vi "WindowBuild.vi"(7 "Init":bool, 8 "error in (no error)":errorcluster, 11 "Fitter in":refnum<class "FitterBase.lvclass">) -> (0 "error out":errorcluster, 2 "Timeout":bool, 3 "Fitter out":refnum<class "FitterBase.lvclass">)   [LabVIEW 2018, in "AnalysisPlugins.lvlib" / "FitterBase.lvclass"]
uses:
  FitterBaseClass/FitterBase.lvclass
  X:/Projects/PMUCal/Modules/Analysis/AnalysisPlugins/AnalysisPluginBaseClass/AnalysisPluginsBase.lvclass
  Typedefs/SampleDataInput.ctl
  FitterBaseClass/Typedefs/clAnalysisConfig.ctl
  AnalysisPluginsBase.lvclass/AnalysisPluginsBase.ctl
  FitterBaseClass/Typedefs/Wvfrm_ref.ctl
  Accessors/Read SensorQue.vi
  Accessors/Read Duration.vi
  Accessors/Read Window.vi
  Accessors/Read AnalysisConfig.vi
  Accessors/Read AnalysisTime.vi
  Accessors/Read SampleDataQueName.vi
  Accessors/Write Window.vi
  <vilib>/Utility/error.llb/Error Cluster From Error Code.vi
  <vilib>/ErrorRing/Error Ring.xnode
  AnalysisPluginsBase.lvclass
panel:
  out "T0":timestamp format="%^<%.3X\n%x>T"
  out "Continue":bool
  out "Valid":bool
  out "SensorTime":timestamp format="%^<%.3X\n%x>T"
  out "WindowTime":timestamp format="%^<%.3X\n%x>T"
  out "SampleTime":timestamp format="%^<%.3X\n%x>T"
  out "SampleData":dbl[][](graph)
  out "Window":dbl[][](graph)
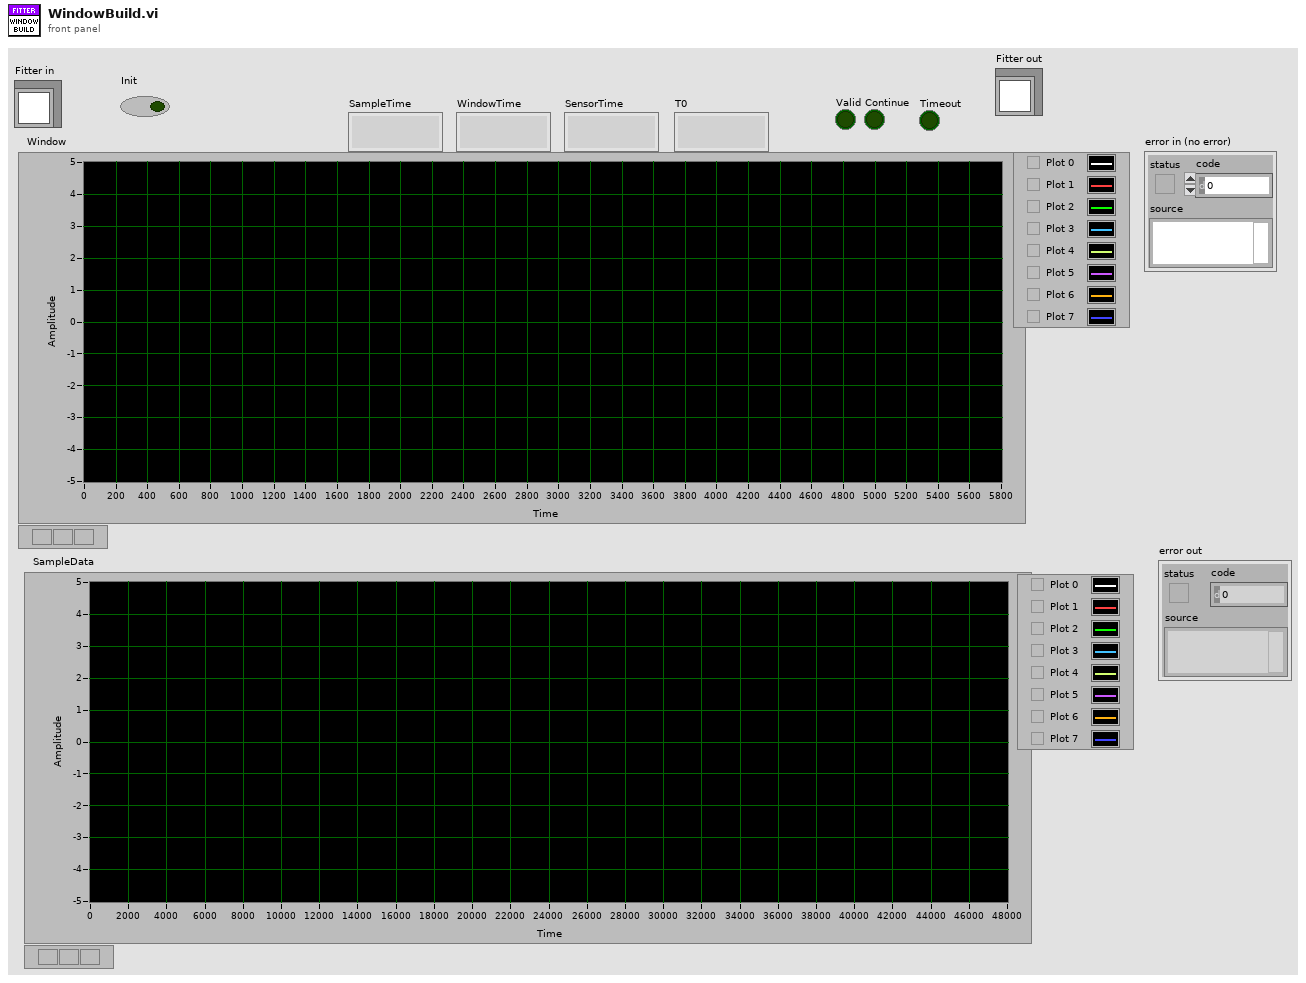
[diagram p1: front panel]
types:
  T1 = typedef "AnalysisPlugins.lvlib/FitterBase.lvclass/clAnalysisConfig.ctl" = cluster{"F0":u32, "SettlingTime":dbl, "AnalysisCycles":dbl, "SampleRate":dbl, "NumChannels":u32, "TsOffset":enum16{"start", "middle", "end"}}
  T2 = typedef "AnalysisPlugins.lvlib/AnalysisPluginsBase.lvclass/SampleDataInput.ctl" = waveform(dbl)[]
  T3 = typedef "AnalysisPlugins.lvlib/FitterBase.lvclass/Wvfrm_ref.ctl" = cluster{"t0":timestamp, "dt":dbl, "attributes":variant, "Y_ref":refnum<data-value>}
  T4 = typedef "AnalysisPlugins.lvlib/AnalysisPluginsBase.lvclass/clWindowData.ctl" = cluster{"Timestamp":ext, "Samples":dbl[][], "Window Valid":bool, "T0":ext}
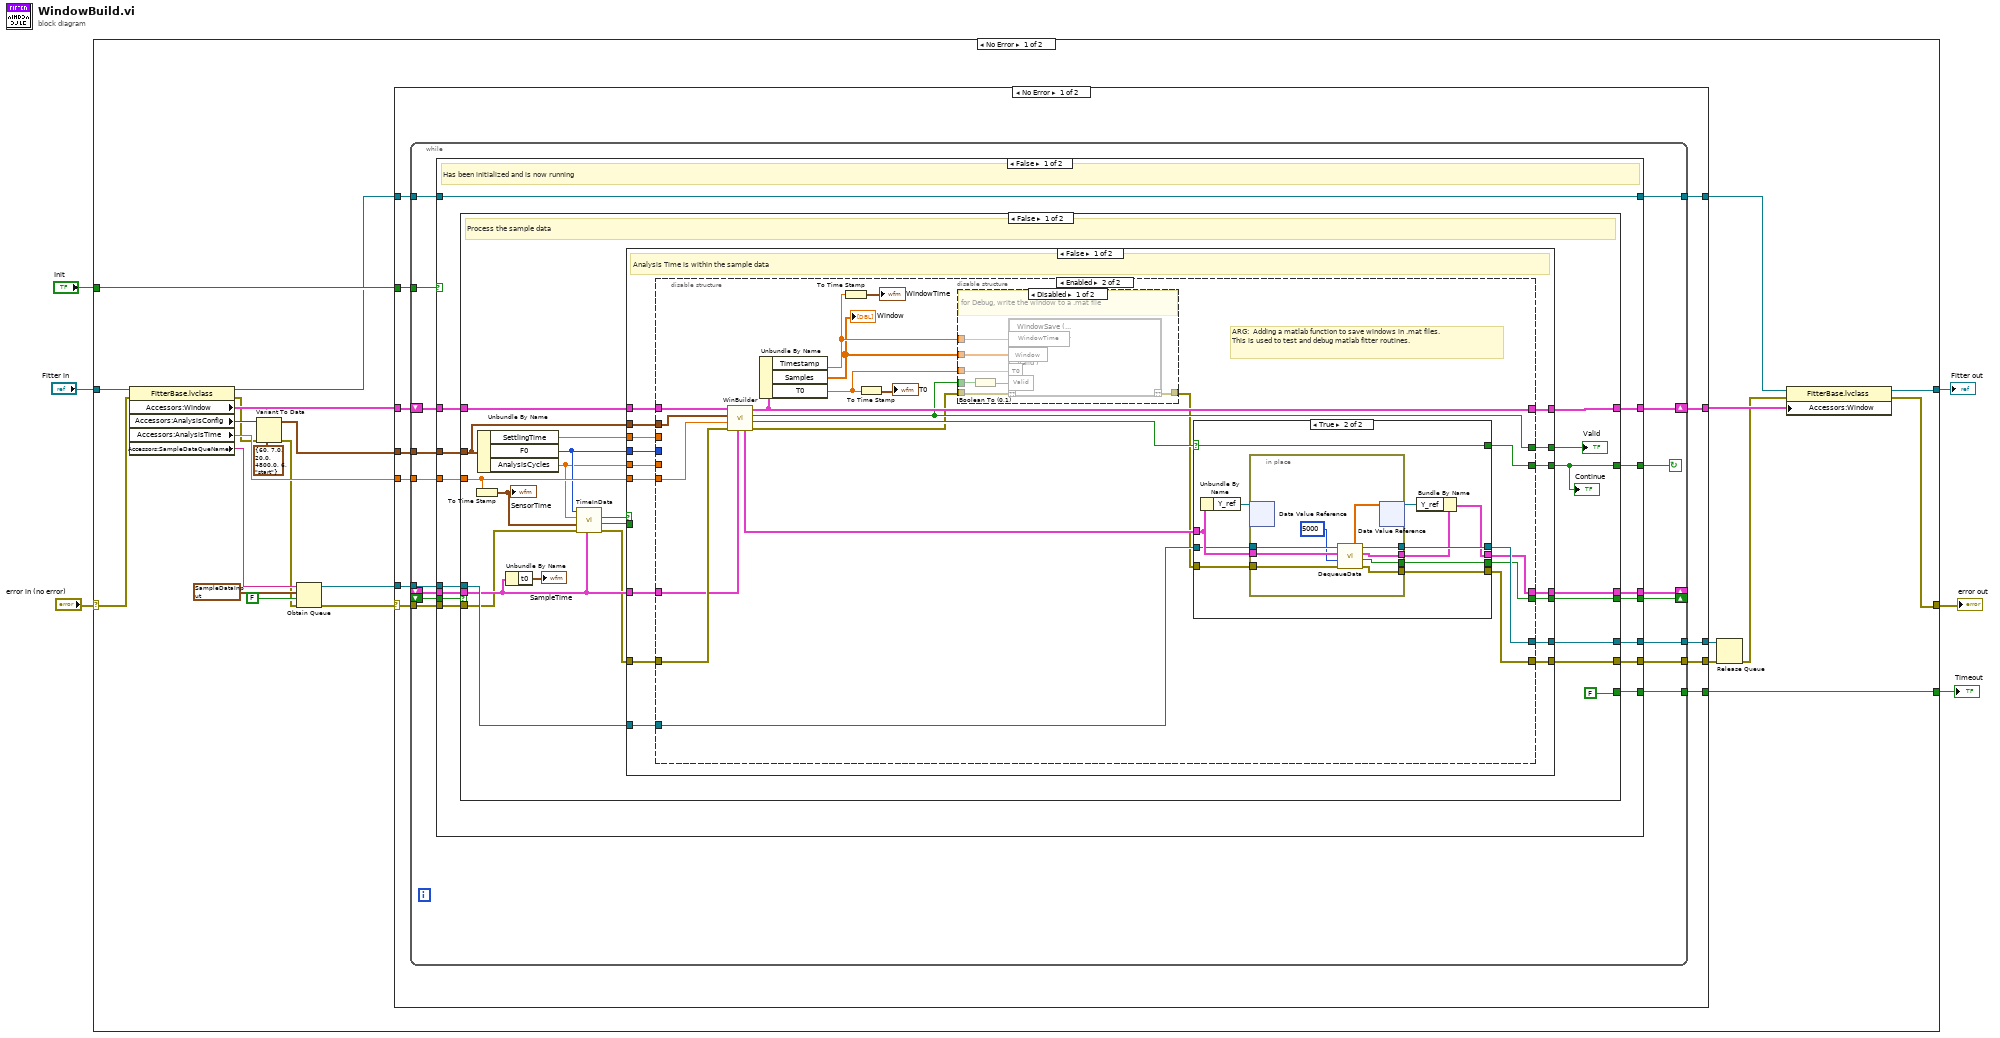
[diagram p0: block diagram]
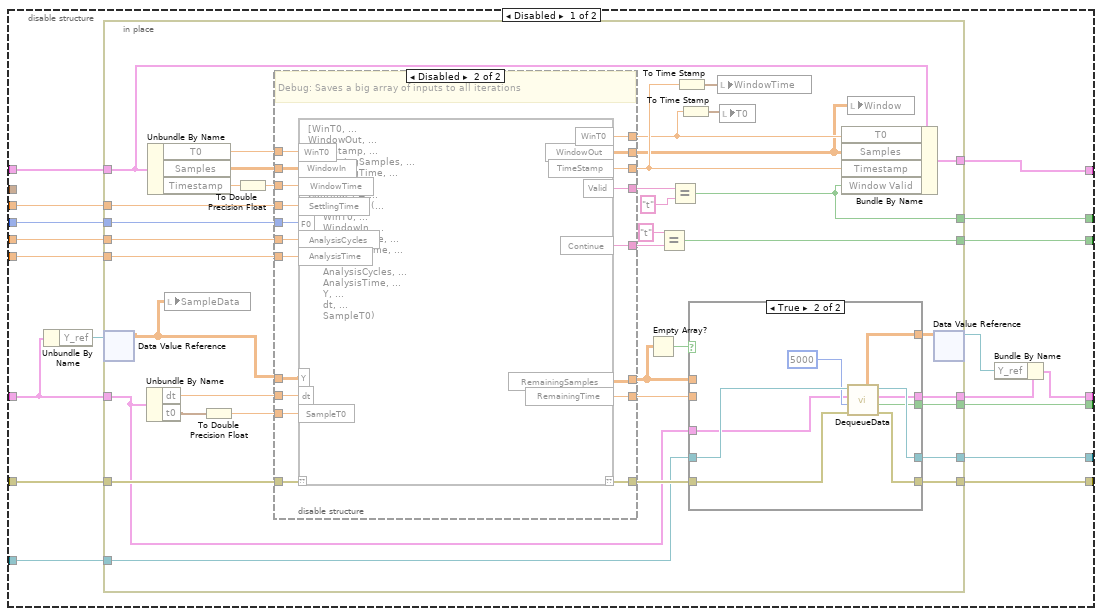
[diagram p2: hidden frame]
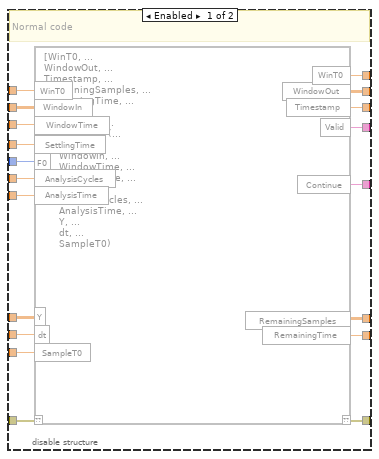
[diagram p3: hidden frame]
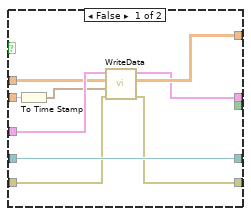
[diagram p4: hidden frame]
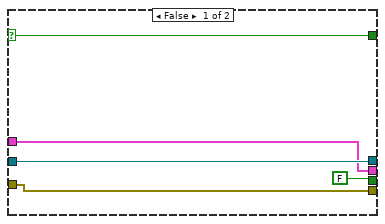
[diagram p6: hidden frame]
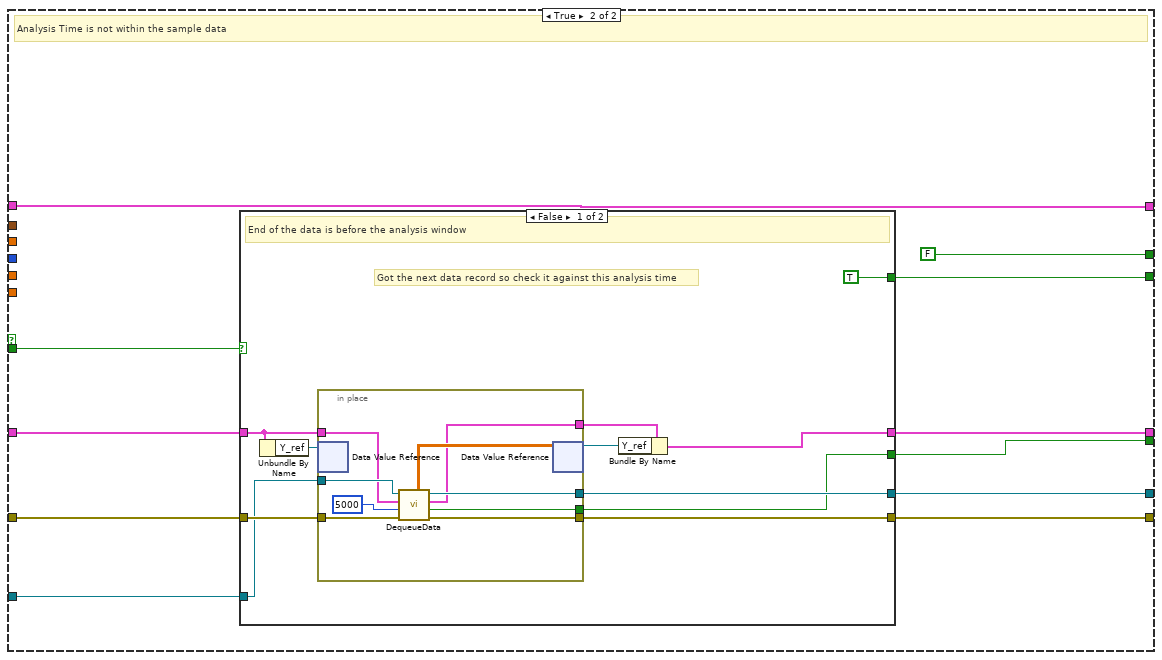
[diagram p7: hidden frame]
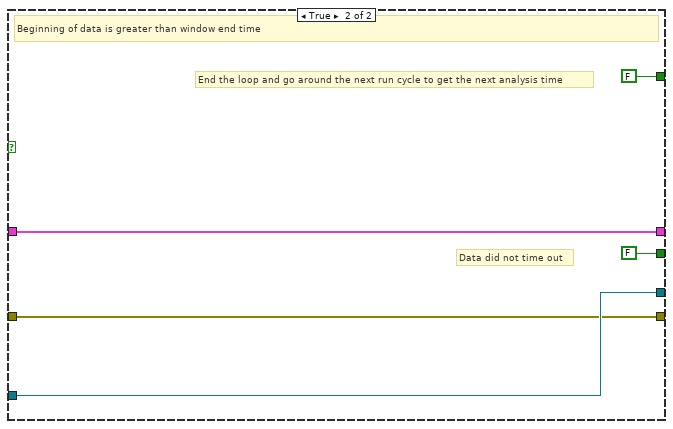
[diagram p8: hidden frame]
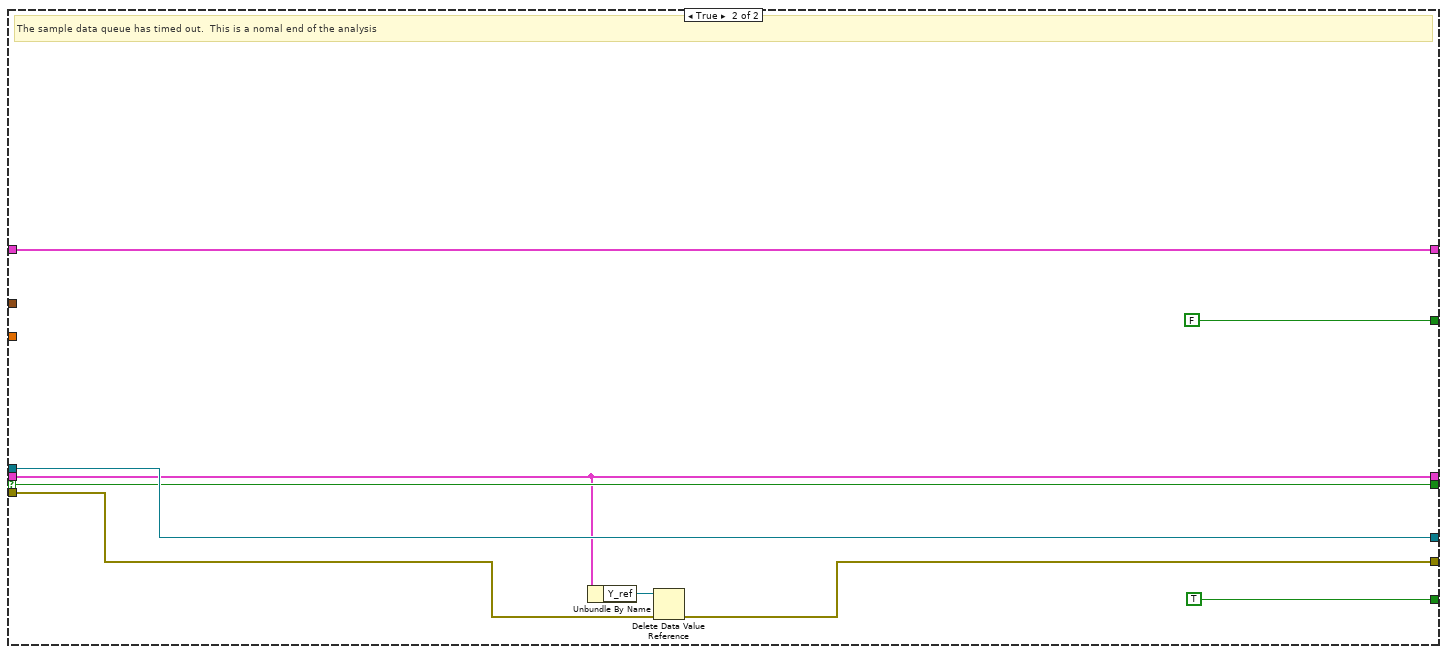
[diagram p9: hidden frame]
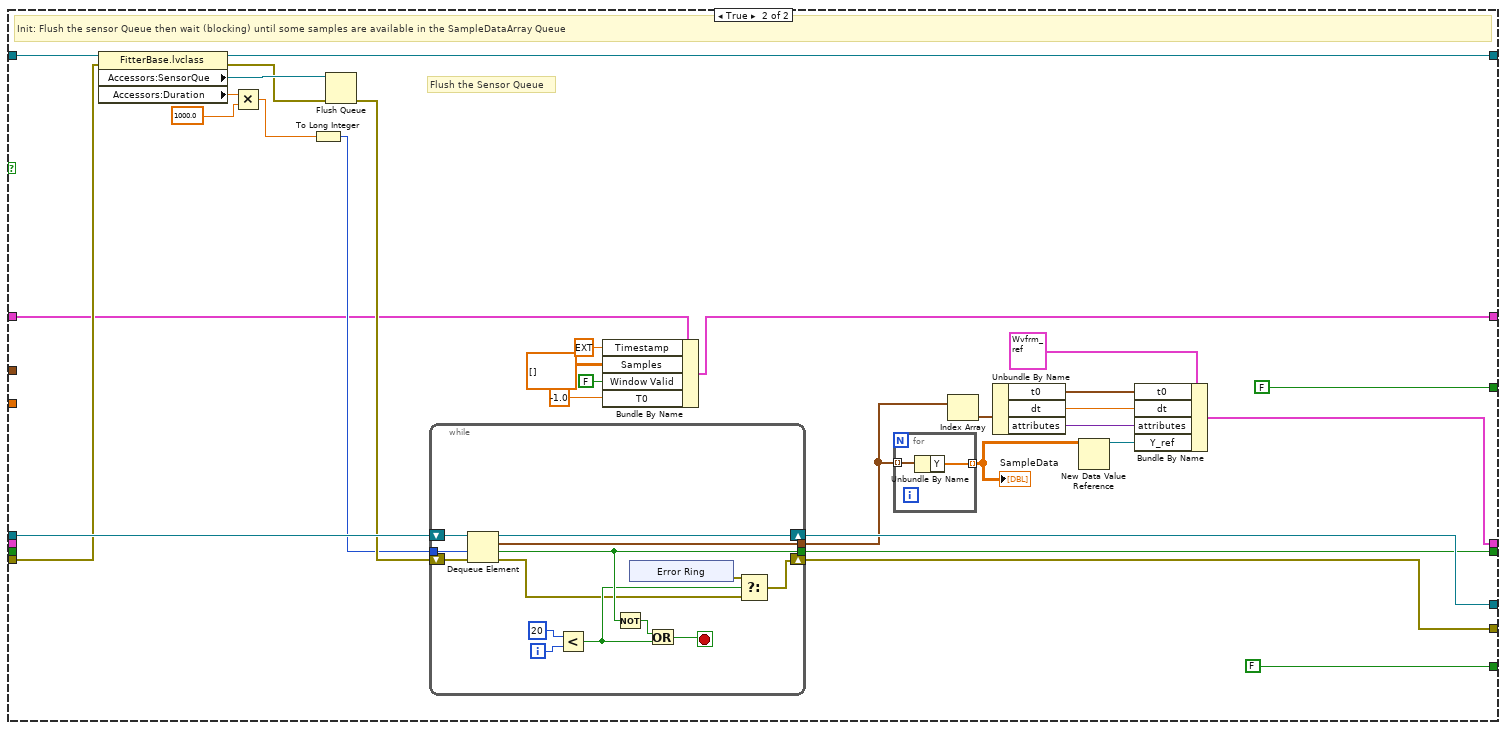
[diagram p10: hidden frame]
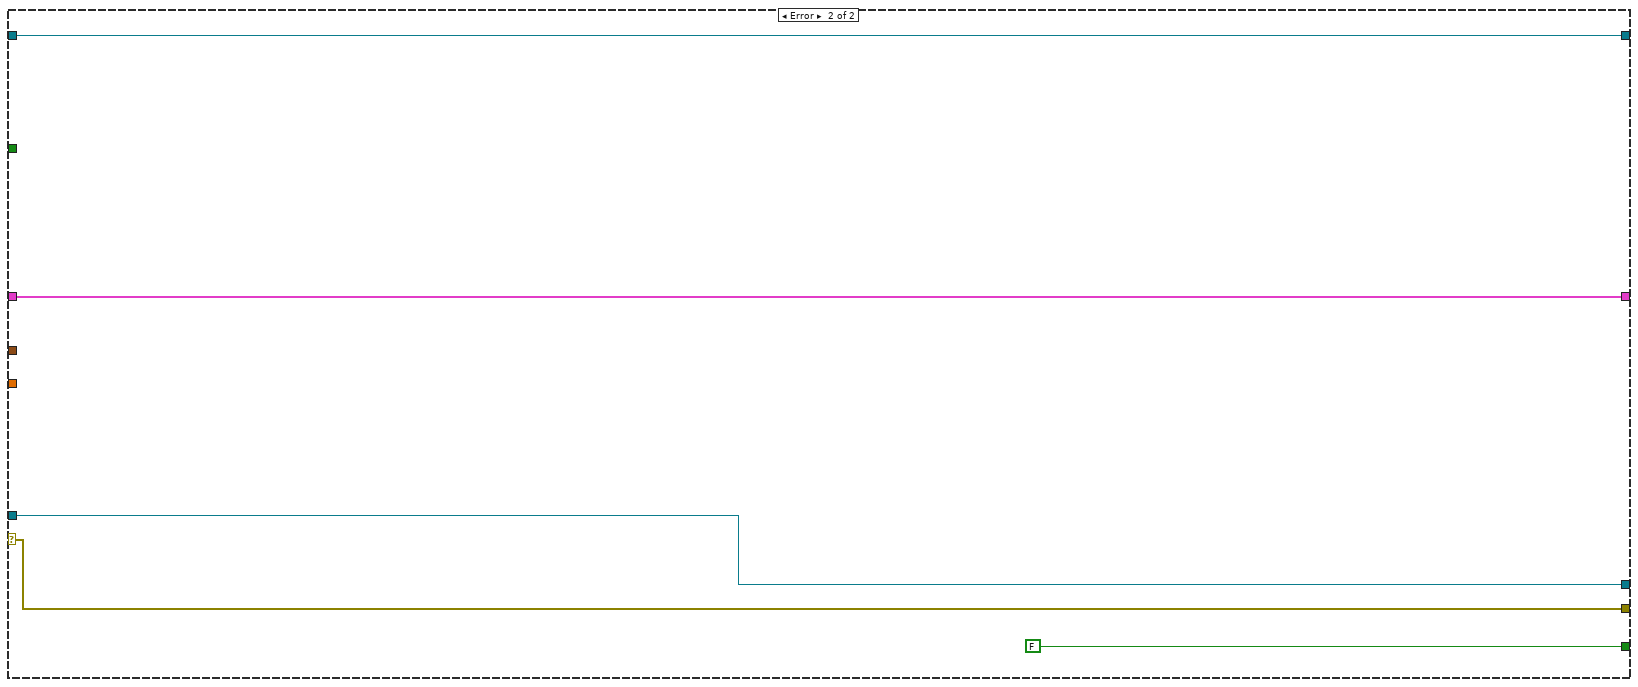
[diagram p11: hidden frame]
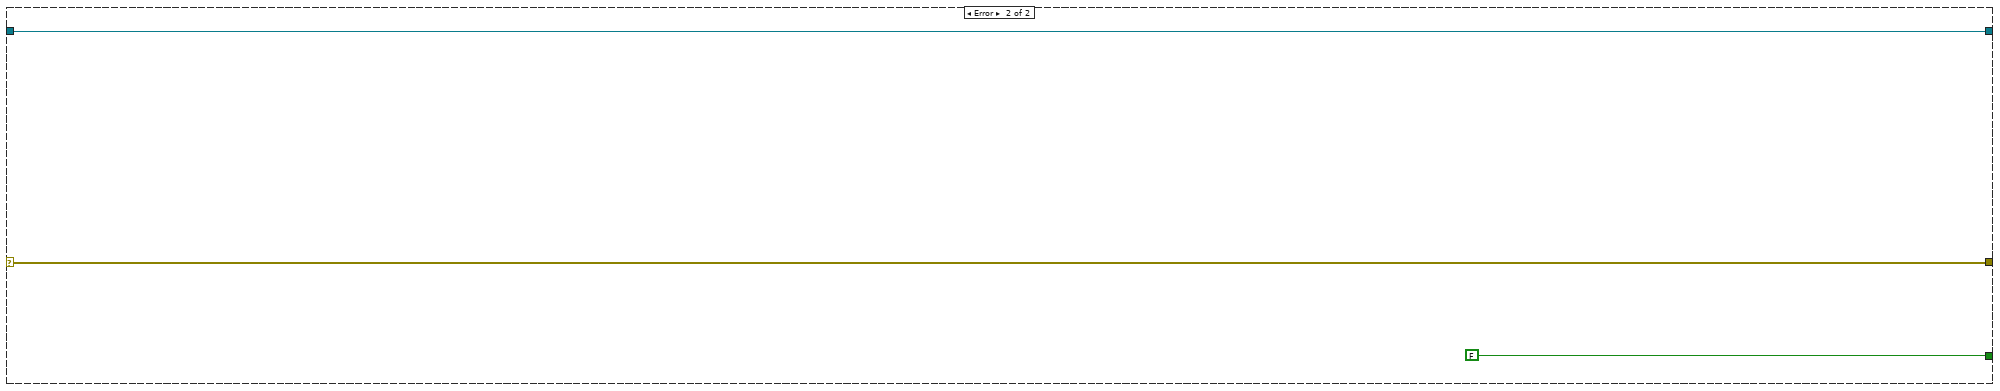
[diagram p12: hidden frame]
diagram:
  n1 = case shown="No Error" "error in (no error)" {
    selector: "error in (no error)" -> [w15 w382]
    tunnel: [w28 w382] -> w5
    tunnel: [w29 w381] -> w3
    tunnel: "Fitter in" -> [w30 w381]
    tunnel: [w18 FALSE] -> w2
    tunnel: "Init" -> [w10 _]
    frame No Error {
      n2 = property class="FitterBase.lvclass"(reference=w30, error in=w15) -> (reference out=w9:refnum<class "FitterBase.lvclass">, error out=w14:errorcluster, "Accessors:Window"=w24:T4, "Accessors:AnalysisConfig"=w17:variant, "Accessors:AnalysisTime"=w25:dbl, "Accessors:SampleDataQueName"=w26:string)
      n3 = Variant To Data(error in=w14, type=T1 {"F0"=60, "SettlingTime"=7.0, "AnalysisCycles"=20.0, "SampleRate"=4800.0, "NumChannels"=6, "TsOffset"=enum."start"} ("clAnalysisConfig"), Variant=w17) -> (data=w7:T1, error out=w13:errorcluster)
      n4 = Obtain Queue(name (unnamed)=w26, element data type=T2 [{"t0"=timestamp(0 s since 1904-01-01), "dt"=1.0, "Y"=[]}] ("clSampleDataArray"), create if not found? (T)=FALSE, error in (no error)=w13) -> (queue out=w12:refnum<queue>, error out=w11:errorcluster)  [unwired: 1 in, 1 out]
      n5 = case shown="No Error" w11 {
        selector: w11 -> [w41 w379]
        tunnel: w25 -> [w42 _]
        tunnel: w12 -> [w40 w378]
        tunnel: w24 -> [w39 w377]
        tunnel: [w38 w377] -> w23
        tunnel: [w37 w379] -> w22
        tunnel: [w36 w378] -> w20
        tunnel: [w35 FALSE] -> w18
        tunnel: w10 -> [w34 _]
        tunnel: w9 -> [w33 w375]
        tunnel: [w32 w375] -> w8
        tunnel: w7 -> [w31 _]
        frame No Error {
          n6 = while {
            tunnel: w42 -> [w59]
            tunnel: w41 -> [w55]
            tunnel: w40 -> [w53]
            shift-right: [w56] -> w38
            shift-left: w39 -> [w57]
            tunnel: [w54] -> w37
            tunnel: [w52] -> w36
            tunnel: [w51] -> w35
            shift-right: [w44] -> _
            shift-left: _ -> [w50]
            shift-right: [w48] -> _
            shift-left: _ -> [w49]
            tunnel: w34 -> [w47]
            tunnel: w33 -> [w46]
            tunnel: [w45] -> w32
            tunnel: w31 -> [w43]
            stop <- w58 continue-if-true
            n7 = case shown="False" w47 {
              tunnel: w50 -> [w61 _]
              tunnel: w59 -> [w74 _]
              tunnel: [w73 FALSE] -> w58
              tunnel: w57 -> [w72 w329]
              tunnel: [w71 w324] -> w56
              tunnel: w49 -> [w70 _]
              tunnel: w55 -> [w69 w345]
              tunnel: [w68 w341] -> w54
              tunnel: w53 -> [w67 w354]
              tunnel: [w66 w353] -> w52
              tunnel: [w65 FALSE] -> w51
              tunnel: [w64 w335] -> w44
              tunnel: [w63 w352] -> w48
              tunnel: w46 -> [w62 w349]
              tunnel: [w62 w346] -> w45
              tunnel: w43 -> [w60 _]
              frame False {
                # "Has been initialized and is now running"
                n8 = case shown="False" w70 {
                  selector: w70 -> [_ w319]
                  tunnel: w74 -> [w89 _]
                  tunnel: [w96 FALSE] -> w73
                  tunnel: w72 -> [w95 w322]
                  tunnel: [w94 w322] -> w71
                  tunnel: w69 -> [w76 w318]
                  tunnel: [w91 w317] -> w68
                  tunnel: w67 -> [w92 w321]
                  tunnel: [w90 w321] -> w66
                  tunnel: [FALSE TRUE] -> w65
                  tunnel: [w81 w316] -> w64
                  tunnel: [w87 w319] -> w63
                  tunnel: w61 -> [w82 w316]
                  tunnel: w60 -> [w77 _]
                  frame False {
                    # "Process the sample data"
                    n9 = To Time Stamp(1:w89) -> (0:w86:timestamp)
                    "SensorTime" <- w86
                    n10 = Unbundle By Name(w77) -> ("SettlingTime"=w80:dbl, "F0"=w79:u32, "AnalysisCycles"=w78:dbl)
                    n11 = Unbundle By Name(w82) -> ("t0"=→"SampleTime":timestamp)
                    n12 = call "TimeInData.vi"("Wvfrm_ref"=w82, "error in (no error)"=w76, "SensorTime"=w86, "AnalysisCycles"=w78, "F0"=w79) -> ("error out"=w75:errorcluster, "AnalysisFirst"=w84:bool, "NoDataInWindow"=w85:bool)  [unwired: 4 in]
                    n13 = case shown="False" w85 {
                      tunnel: w79 -> [w112 _]
                      tunnel: w78 -> [w111 _]
                      tunnel: [w110 w280] -> w96
                      tunnel: w95 -> [w109 w289]
                      tunnel: [w108 w289] -> w94
                      tunnel: [w107 FALSE] -> w93
                      tunnel: w92 -> [w106 w284]
                      tunnel: [w105 w281] -> w91
                      tunnel: [w104 w283] -> w90
                      tunnel: w75 -> [w103 w282]
                      tunnel: w89 -> [w102 _]
                      tunnel: w80 -> [w101 _]
                      tunnel: [w98 w279] -> w81
                      tunnel: [w100 w285] -> w87
                      tunnel: w82 -> [w99 w286]
                      tunnel: w84 -> [_ w287]
                      tunnel: w77 -> [w97 _]
                      frame False {
                        # "Analysis Time is within the sample data"
                        n14 = disable-structure shown="Enabled" {
                          disable-tunnel: w112 -> [w130 _]
                          disable-tunnel: w111 -> [w129 _]
                          disable-tunnel: [w128 w231] -> w110
                          disable-tunnel: w109 -> [w127 w245]
                          disable-tunnel: [w126 w240] -> w108
                          disable-tunnel: [w125 w227] -> w107
                          disable-tunnel: w106 -> [w124 w234]
                          disable-tunnel: [w123 w232] -> w105
                          disable-tunnel: [w122 w235] -> w104
                          disable-tunnel: w103 -> [w121 w243]
                          disable-tunnel: w102 -> [w120 w242]
                          disable-tunnel: w101 -> [w119 _]
                          disable-tunnel: [w118 w230] -> w100
                          disable-tunnel: w99 -> [w117 w241]
                          disable-tunnel: [w113 w233] -> w98
                          disable-tunnel: w97 -> [_ w244]
                          frame Disabled {
                            n15 = Unbundle By Name(w117) -> ("Y_ref"=w116:refnum<data-value>)
                            n16 = in-place {
                              in-place-border: w130 -> [w167]
                              in-place-border: w129 -> [w166]
                              in-place-border: [w165] -> w128
                              in-place-border: w127 -> [w164]
                              in-place-border: [w163] -> w126
                              in-place-border: [w157] -> w125
                              in-place-border: w124 -> [w154]
                              in-place-border: [w153] -> w123
                              in-place-border: [w151] -> w122
                              in-place-border: w121 -> [w150]
                              in-place-border: w120 -> [w148]
                              in-place-border: w119 -> [w146]
                              in-place-border: [w144] -> w118
                              in-place-border: w117 -> [w142]
                              in-place-border: [w143] -> w115
                              n17 = in-place-dvr #1(w116) -> (w136:dbl[][])  [unwired: 1 out]
                              n18 = Unbundle By Name(w142) -> ("dt"=w139:dbl, "t0"=w138:timestamp)
                              n19 = Unbundle By Name(w164) -> ("T0"=w145:ext, "Samples"=w162:dbl[][], "Timestamp"=w149:ext)
                              n20 = local write "SampleData"(w136) -> ()
                              n21 = To Double Precision Float(number=w138) -> (double precision float=w137:dbl)
                              n22 = To Double Precision Float(number=w149) -> (double precision float=w156:dbl)
                              n23 = disable-structure shown="Disabled" {
                                disable-tunnel: w167 -> [w186 w203]
                                disable-tunnel: w166 -> [w185 w202]
                                disable-tunnel: w148 -> [w184 w201]
                                disable-tunnel: w162 -> [w183 w205]
                                disable-tunnel: [w182 w196] -> w161
                                disable-tunnel: [w181 w199] -> w131
                                disable-tunnel: [w180 w198] -> w134
                                disable-tunnel: [w179 w197] -> w159
                                disable-tunnel: w150 -> [w178 w193]
                                disable-tunnel: w136 -> [w177 w200]
                                disable-tunnel: w156 -> [w176 w204]
                                disable-tunnel: [w175 w194] -> w155
                                disable-tunnel: [w174 w195] -> w147
                                disable-tunnel: w146 -> [w172 w192]
                                disable-tunnel: w145 -> [w173 w191]
                                disable-tunnel: [w171 w190] -> w132
                                disable-tunnel: [w170 w189] -> w140
                                disable-tunnel: w139 -> [w169 w187]
                                disable-tunnel: w137 -> [w168 w188]
                                frame Enabled {
                                # "Normal code"
                                n24 = script code="[WinT0, ...\nWindowOut, ...\nTimestamp, ...\nRemainingSamples, ...\nRemainingTime, ...\nValid, ...\nContinue] = ...\nWindowBuild (...\n     WinT0, ...\n     WindowIn, ...\n     WindowTime, ...\n     SettlingTime, ...\n      F0, ...\n     AnalysisCycles, ...\n     AnalysisTime, ...\n     Y, ...\n     dt, ...\n     SampleT0)"("??"=w178, "F0"=w186, "AnalysisCycles"=w185, "AnalysisTime"=w184, "WindowTime"=w176, "Y"=w177, "dt"=w169, "SampleT0"=w168, "WindowIn"=w183, "WinT0"=w173, "SettlingTime"=w172) -> ("??"=w175:errorcluster, "Continue"=w182:string, "WindowOut"=w181:dbl[][], "Timestamp"=w180:dbl, "Valid"=w179:string, "RemainingSamples"=w174:dbl[][], "RemainingTime"=w170:dbl, "WinT0"=w171:dbl)
                                }
                                frame Disabled {
                                # "Debug: Saves a big array of inputs to all iterations"
                                n25 = script code="[WinT0, ...\nWindowOut, ...\nTimeStamp, ...\nRemainingSamples, ...\nRemainingTime, ...\nValid, ...\nContinue] = ...\nWindowSave (...\n     WinT0, ...\n     WindowIn, ...\n     WindowTime, ...\n      SettlingTime, ...\n      F0, ...\n     AnalysisCycles, ...\n     AnalysisTime, ...\n     Y, ...\n     dt, ...\n     SampleT0)"("??"=w193, "F0"=w203, "AnalysisCycles"=w202, "AnalysisTime"=w201, "WindowTime"=w204, "Y"=w200, "dt"=w187, "SampleT0"=w188, "WindowIn"=w205, "SettlingTime"=w192, "WinT0"=w191) -> ("??"=w194:errorcluster, "Continue"=w196:string, "WindowOut"=w199:dbl[][], "TimeStamp"=w198:dbl, "Valid"=w197:string, "RemainingSamples"=w195:dbl[][], "RemainingTime"=w189:dbl, "WinT0"=w190:dbl)
                                }
                              }
                              n26 = Empty Array?(array=w147) -> (empty?=w152:bool)
                              n27 = Equal?(x="t", y=w161) -> (x = y?=w165:bool)
                              n28 = Equal?(x=w159, y="t") -> (x = y?=w157:bool)
                              n29 = To Time Stamp(1:w134) -> (0:w135:timestamp)
                              n30 = To Time Stamp(1:w132) -> (0:w133:timestamp)
                              n31 = case shown="True" w152 {
                                tunnel: w155 -> [w208 w220]
                                tunnel: w154 -> [w214 w223]
                                tunnel: [w207 w218] -> w153
                                tunnel: [w214 w222] -> w151
                                tunnel: w147 -> [w211 _]
                                tunnel: [w209 w221] -> w143
                                tunnel: [_ w219] -> w144
                                tunnel: w142 -> [w212 w216]
                                tunnel: [w210 w215] -> w141
                                tunnel: w140 -> [w213 _]
                                frame False {
                                n32 = To Time Stamp(1:w213) -> (0:w206:timestamp)
                                n33 = call "WriteData.vi"("error in (no error)"=w208, "t0"=w206, "data value"=w211, "Wvfrm_ref"=w212) -> ("error out"=w207:errorcluster, "data value"=w210:dbl[][], "Wvfrm_ref"=w209:T3)  [unwired: 5 in]
                                }
                                frame True {
                                n34 = call "DequeueData.vi"("error in (no error)"=w220, "timeout in ms (-1)"=5000, "DataIn"=w216, "queue in"=w223) -> ("error out"=w218:errorcluster, "timed out?"=w219:bool, "Data Out"=w221:T3, "queue out"=w222:refnum<queue>, "Y"=w215:dbl[][])  [unwired: 3 in]
                                }
                              }
                              n35 = local write "WindowTime"(w135) -> ()
                              n36 = local write "T0"(w133) -> ()
                              n37 = Bundle By Name(cluster=w164, "T0"=w132, "Samples"=w131, "Timestamp"=w134, "Window Valid"=w157) -> (w163:T4)
                              n38 = local write "Window"(w131) -> ()
                              n39 = in-place-dvr #1(w141) -> (w114:refnum<data-value>)  [unwired: 1 out]
                            }
                            n40 = Bundle By Name(cluster=w115, "Y_ref"=w114) -> (w113:T3)
                          }
                          frame Enabled {
                            # "ARG:  Adding a matlab function to save windows in .mat files.\nThis is used to test and debug matlab fitter routines."
                            n41 = call "WinBuilder.vi"("Wvfrm_ref"=w241, "error in (no error)"=w243, "AnalysisTime"=w242, "clAnalysisConfig"=w244, "Window"=w245) -> ("error out"=w225:errorcluster, "Continue"=w237:bool, "Valid"=w227:bool, "Window"=w240:T4, "Wvfrm_ref"=w236:T3)  [unwired: 2 in]
                            n42 = Unbundle By Name(w240) -> ("Timestamp"=w229:ext, "Samples"=w228:dbl[][], "T0"=w226:ext)
                            "Window" <- w228
                            n43 = To Time Stamp(1:w229) -> (0:→"WindowTime":timestamp)
                            n44 = To Time Stamp(1:w226) -> (0:→"T0":timestamp)
                            n45 = disable-structure shown="Disabled" {
                              disable-tunnel: w225 -> [w252 w253]
                              disable-tunnel: w229 -> [w251 _]
                              disable-tunnel: w228 -> [w250 _]
                              disable-tunnel: w227 -> [w249 _]
                              disable-tunnel: w226 -> [w247 _]
                              disable-tunnel: [w246 w253] -> w224
                              frame Disabled {
                                # "for Debug, write the window to a .mat file"
                                n46 = Boolean To (0,1)(Boolean=w249) -> (0, 1=w248:i16)
                                n47 = script code="WindowSave (...\nWindowTime, ...\nWindow, ...\nT0, ...\nValid )"("??"=w252, "WindowTime"=w251, "Window"=w250, "T0"=w247, "Valid"=w248) -> ("??"=w246:errorcluster)
                              }
                              frame Enabled {
                              }
                            }
                            n48 = case shown="True" w237 {
                              selector: w237 -> [w255 w263]
                              tunnel: w234 -> [w258 w267]
                              tunnel: w236 -> [w257 w269]
                              tunnel: w224 -> [w256 w266]
                              tunnel: [w258 w265] -> w235
                              tunnel: [w257 w260] -> w233
                              tunnel: [w256 w264] -> w232
                              tunnel: [w255 w263] -> w231
                              tunnel: [FALSE w262] -> w230
                              frame False {
                              }
                              frame True {
                                n49 = Unbundle By Name(w269) -> ("Y_ref"=w268:refnum<data-value>)
                                n50 = in-place {
                                in-place-border: w269 -> [w277]
                                in-place-border: w267 -> [w278]
                                in-place-border: w266 -> [w275]
                                in-place-border: [w273] -> w265
                                in-place-border: [w272] -> w261
                                in-place-border: [w271] -> w262
                                in-place-border: [w270] -> w264
                                n51 = in-place-dvr #2(w268) -> ()  [unwired: 2 out]
                                n52 = call "DequeueData.vi"("error in (no error)"=w275, "timeout in ms (-1)"=5000, "DataIn"=w277, "queue in"=w278) -> ("error out"=w270:errorcluster, "timed out?"=w271:bool, "Data Out"=w272:T3, "queue out"=w273:refnum<queue>, "Y"=w274:dbl[][])  [unwired: 3 in]
                                n53 = in-place-dvr #2(w274) -> (w259:refnum<data-value>)  [unwired: 1 out]
                                }
                                n54 = Bundle By Name(cluster=w261, "Y_ref"=w259) -> (w260:T3)
                              }
                            }
                          }
                        }
                      }
                      frame True {
                        # "Analysis Time is not within the sample data"
                        n55 = case shown="False" w287 {
                          tunnel: w286 -> [w294 w314]
                          tunnel: [w290 w314] -> w279
                          tunnel: [w295 FALSE] -> w285
                          tunnel: w284 -> [w298 w312]
                          tunnel: [w297 w312] -> w283
                          tunnel: w282 -> [w299 w311]
                          tunnel: [w296 w311] -> w281
                          tunnel: [TRUE FALSE] -> w280
                          frame False {
                            # "Got the next data record so check it against this analysis time"
                            # "End of the data is before the analysis window"
                            n56 = Unbundle By Name(w294) -> ("Y_ref"=w293:refnum<data-value>)
                            n57 = in-place {
                              in-place-border: w299 -> [w309]
                              in-place-border: w298 -> [w307]
                              in-place-border: w294 -> [w306]
                              in-place-border: [w305] -> w297
                              in-place-border: [w304] -> w296
                              in-place-border: [w303] -> w295
                              in-place-border: [w301] -> w292
                              n58 = in-place-dvr #3(w293) -> ()  [unwired: 2 out]
                              n59 = call "DequeueData.vi"("error in (no error)"=w309, "timeout in ms (-1)"=5000, "DataIn"=w306, "queue in"=w307) -> ("error out"=w304:errorcluster, "timed out?"=w303:bool, "Data Out"=w301:T3, "queue out"=w305:refnum<queue>, "Y"=w302:dbl[][])  [unwired: 3 in]
                              n60 = in-place-dvr #3(w302) -> (w291:refnum<data-value>)  [unwired: 1 out]
                            }
                            n61 = Bundle By Name(cluster=w292, "Y_ref"=w291) -> (w290:T3)
                          }
                          frame True {
                            # "End the loop and go around the next run cycle to get the next analysis time"
                            # "Data did not time out"
                            # "Beginning of data is greater than window end time"
                          }
                        }
                      }
                    }
                    "Valid" <- w93
                    "Continue" <- w96
                  }
                  frame True {
                    # "The sample data queue has timed out.  This is a nomal end of the analysis"
                    n62 = Unbundle By Name(w316) -> ("Y_ref"=w315:refnum<data-value>)
                    n63 = Delete Data Value Reference(data value reference=w315, error in=w318) -> (error out=w317:errorcluster)  [unwired: 1 out]
                  }
                }
              }
              frame True {
                # "Flush the Sensor Queue"
                # "Init: Flush the sensor Queue then wait (blocking) until some samples are available in the SampleDataArray Queue"
                n64 = property class="FitterBase.lvclass"(reference=w349, error in=w345) -> (reference out=w346:refnum<class "FitterBase.lvclass">, error out=w347:errorcluster, "Accessors:SensorQue"=w348:refnum<queue>, "Accessors:Duration"=w344:dbl)
                n65 = Multiply(x=w344, y=1000.0) -> (x*y=w330:dbl)
                n66 = To Long Integer(number=w330) -> (32bit integer=w331:i32)
                n67 = Flush Queue(queue=w348, error in (no error)=w347) -> (error out=w342:errorcluster)  [unwired: 2 out]
                n68 = while {
                  tunnel: [w361] -> w352
                  tunnel: [w365] -> w334
                  tunnel: w331 -> [w364]
                  shift-right: [w367] -> w353
                  shift-left: w354 -> [w368]
                  shift-right: [w355] -> w341
                  shift-left: w342 -> [w366]
                  i -> [w363]
                  stop <- w359 stop-if-true
                  n69 = Dequeue Element(queue=w368, timeout in ms (-1)=w364, error in (no error)=w366) -> (queue out=w367:refnum<queue>, element=w365:T2, timed out?=w361:bool, error out=w357:errorcluster)
                  n70 = Less?(x=20 ("timeout in ms (-1)"), y=w363) -> (x < y?=w358:bool)
                  n71 = Not(x=w361) -> (.not. x?=w360:bool)
                  n72 = xnode "Error Ring"() -> ("error out"=w356:errorcluster)
                  n73 = Or(x=w360, y=w358) -> (x .or. y?=w359:bool)
                  n74 = Select(t=w356, s=w358, f=w357) -> (s? t:f=w355:errorcluster)
                }
                n75 = Bundle By Name(cluster=w329, "Timestamp"=ext 0.0, "Samples"=dbl[][] [], "Window Valid"=FALSE, "T0"=-1.0) -> (w324:T4)
                n76 = for {
                  tunnel: w334 -> [w374] mode=indexing
                  tunnel: [w373] -> w332 mode=indexing
                  n77 = Unbundle By Name(w374) -> ("Y"=w373:dbl[])
                }
                "SampleData" <- w332
                n78 = Index Array(array=w334) -> (element=w340:waveform(dbl))  [unwired: 1 in]
                n79 = Unbundle By Name(w340) -> ("t0"=w338:timestamp, "dt"=w337:dbl, "attributes"=w336:variant)
                n80 = New Data Value Reference(data value=w332) -> (data value reference=w333:refnum<data-value>)  [unwired: 1 in, 1 out]
                n81 = Bundle By Name(cluster=T3 {"t0"=timestamp(0 s since 1904-01-01), "dt"=1.0, "attributes"=variant, "Y_ref"=refnum} ("Wvfrm_ref"), "t0"=w338, "dt"=w337, "attributes"=w336, "Y_ref"=w333) -> (w335:T3)
              }
            }
          }
        }
        frame Error {
        }
      }
      n82 = Release Queue(queue=w20, error in (no error)=w22) -> (error out=w21:errorcluster)  [unwired: 1 in, 2 out]
      n83 = property class="FitterBase.lvclass"(reference=w8, error in=w21, "Accessors:Window"=w23) -> (reference out=w29:refnum<class "FitterBase.lvclass">, error out=w28:errorcluster)
    }
    frame Error {
    }
  }
  "error out" <- w5
  "Fitter out" <- w3
  "Timeout" <- w2
